vi "Swept H(f) from IIR cluster.vi"(6 "Sweep specs":T2={"Fstart"=1e-06, "Fstop"=0.4, "# points"=100, "type"=1} {"type" items=["linear", "exponential"]; "Fstop" format="%.2p"; "Fstart" format="%.2p"}, 9 "Fs":dbl=1.0 format="%.3p", 11 "IIR Filter Cluster":T1 {"Forward Coefficients" format="%.4f"; "Reverse Coefficients" format="%.4f"}) -> (2 "Phase (degrees)":cluster{dbl[], dbl[]}(graph)={[1e-06, 1.1391645578553926e-06, 1.2976958898738721e-06, 1.47828916461893e-06, 1.684014622595541e-06, 1.9183697729710654e-06, 2.1853388542297337e-06, 2.489460569642825e-06, 2.8359052491156023e-06, 3.230562749228562e-06, 3.6801425858490564e-06, 4.1922880016535415e-06, 4.775705907806124e-06, 5.440314908913349e-06, 6.197413927806377e-06, 7.059874296916403e-06, 8.042358581961425e-06, 9.161569858134609e-06, 1.0436535676703204e-05, 1.1888931549693636e-05, 1.3543449452179778e-05, 1.5428217607029237e-05, 1.7575278688808244e-05, 2.002113457672155e-05, 2.2807366917854315e-05, 2.598134405082322e-05, 2.9597026308144866e-05, 3.371588338815227e-05, 3.840793939256846e-05, 4.3752963296271964e-05, 4.984182508826087e-05, 5.6778040639374506e-05, 6.467953156084857e-05, 7.368062997280797e-05, 8.393436226548058e-05, 9.561505067903054e-05, 0.00010892127693109878, 0.00012407925827625992, 0.0001413466933933007, 0.0001610171434837011, 0.0001834250230637487, 0.00020895128529803048, 0.0002380298985298469, 0.000271155224115117, 0.00030889042098927716, 0.000351877019852016, 0.000400845829739195, 0.00045662936240302806, 0.0005201759857256353, 0.0005925660467861364, 0.0006750302386872469, 0.0007689705233931778, 0.0008759839662850192, 0.000997889887641487, 0.001136760792643482, 0.0012949576057390579, 0.0014751698083832116, 0.0016804611625284855, 0.0019143217972049213, 0.002180727543705885, 0.0024842075281287907, 0.002829921170401872, 0.0032237458988464635, 0.0036723770714975667, 0.004183441802930807, 0.004765628631749439, 0.005428835233189849, 0.006184336688086492, 0.007044977168912931, 0.008025388301726034, 0.009142237916353577, 0.010414513413791729, 0.01186384456830111, 0.013514871252113834, 0.015395662334386813, 0.017538192876042673, 0.01997888773321975, 0.022759240811055802, 0.02592652049565079, 0.029534573257156804, 0.03364473908593674, 0.038326894324991166, 0.043660639627698915, 0.04973665323717127, 0.056658232594129186, 0.06454305048195917, 0.0735251555649193, 0.08375725133036026, 0.09541329217893284, 0.10869144079854141, 0.123817437099936, 0.14104843598873648, 0.16067737921930364, 0.18303797565572127, 0.20851037460859584, 0.23752762869926336, 0.2705830561256362, 0.30823862749452124, 0.3511345198037494, 0.40000000000000374], [-1.9375458649467934, -2.206420614039625, -2.512349605053203, -2.860316782462487, -3.2559181849934364, -3.7054091499612234, -4.21574082276718, -4.794577025773823, -5.450278424878941, -6.191835453674648, -7.028724507250726, -7.970653736952076, -9.027156331264258, -10.206982762762935, -11.517243576328537, -12.9622682973866, -14.542184402441919, -16.251294530613507, -18.076446778055725, -19.99574219328411, -21.97806486554142, -23.983974500130337, -25.96836944127362, -27.884943680286753, -29.691867439660662, -31.357509793883324, -32.86468078379547, -34.21203701438905, -35.41200912612372, -36.48566534908234, -37.455944713890034, -38.341281611044664, -39.15155180775962, -39.88750210607899, -40.543640220832486, -41.113376045518294, -41.594444666033596, -41.9925811703799, -42.32208102040144, -42.6030285269283, -42.856196280103276, -43.09747087910708, -43.33383712202392, -43.56239072935225, -43.77275390492707, -43.95203592905604, -44.09055837692053, -44.1862863529227, -44.24637478614913, -44.285282336320996, -44.32014685127728, -44.36510689103546, -44.426634567539026, -44.501577299794185, -44.57862385087098, -44.64266924284485, -44.680502357974596, -44.68575986661503, -44.661355232192065, -44.61850540966146, -44.57270899214032, -44.53813286423849, -44.522440426494676, -44.523933722993824, -44.532042847954976, -44.530983308954184, -44.505254096957685, -44.44498145206778, -44.34916836352415, -44.22566764157143, -44.087881722818125, -43.94937644139832, -43.81835048285295, -43.6939531036865, -43.56577140029595, -43.41665885915146, -43.227865076298286, -42.98459058766059, -42.679934077247935, -42.315778839892594, -41.90027049475206, -41.44276843348109, -40.94806443905276, -40.41192286426785, -39.81951267901921, -39.147248640441994, -38.36731824622104, -37.453191443507, -36.38404639137267, -35.14642919371123, -33.732458269032456, -32.135124592057934, -30.34227788632209, -28.331347333992532, -26.066552278969493, -23.499412451363234, -20.572098548544368, -17.222013665578167, -13.385367266066789, -8.997654066440159]}, 3 "Magnitude (dB)":cluster{dbl[], dbl[]}(graph)={[1e-06, 1.1391645578553926e-06, 1.2976958898738721e-06, 1.47828916461893e-06, 1.684014622595541e-06, 1.9183697729710654e-06, 2.1853388542297337e-06, 2.489460569642825e-06, 2.8359052491156023e-06, 3.230562749228562e-06, 3.6801425858490564e-06, 4.1922880016535415e-06, 4.775705907806124e-06, 5.440314908913349e-06, 6.197413927806377e-06, 7.059874296916403e-06, 8.042358581961425e-06, 9.161569858134609e-06, 1.0436535676703204e-05, 1.1888931549693636e-05, 1.3543449452179778e-05, 1.5428217607029237e-05, 1.7575278688808244e-05, 2.002113457672155e-05, 2.2807366917854315e-05, 2.598134405082322e-05, 2.9597026308144866e-05, 3.371588338815227e-05, 3.840793939256846e-05, 4.3752963296271964e-05, 4.984182508826087e-05, 5.6778040639374506e-05, 6.467953156084857e-05, 7.368062997280797e-05, 8.393436226548058e-05, 9.561505067903054e-05, 0.00010892127693109878, 0.00012407925827625992, 0.0001413466933933007, 0.0001610171434837011, 0.0001834250230637487, 0.00020895128529803048, 0.0002380298985298469, 0.000271155224115117, 0.00030889042098927716, 0.000351877019852016, 0.000400845829739195, 0.00045662936240302806, 0.0005201759857256353, 0.0005925660467861364, 0.0006750302386872469, 0.0007689705233931778, 0.0008759839662850192, 0.000997889887641487, 0.001136760792643482, 0.0012949576057390579, 0.0014751698083832116, 0.0016804611625284855, 0.0019143217972049213, 0.002180727543705885, 0.0024842075281287907, 0.002829921170401872, 0.0032237458988464635, 0.0036723770714975667, 0.004183441802930807, 0.004765628631749439, 0.005428835233189849, 0.006184336688086492, 0.007044977168912931, 0.008025388301726034, 0.009142237916353577, 0.010414513413791729, 0.01186384456830111, 0.013514871252113834, 0.015395662334386813, 0.017538192876042673, 0.01997888773321975, 0.022759240811055802, 0.02592652049565079, 0.029534573257156804, 0.03364473908593674, 0.038326894324991166, 0.043660639627698915, 0.04973665323717127, 0.056658232594129186, 0.06454305048195917, 0.0735251555649193, 0.08375725133036026, 0.09541329217893284, 0.10869144079854141, 0.123817437099936, 0.14104843598873648, 0.16067737921930364, 0.18303797565572127, 0.20851037460859584, 0.23752762869926336, 0.2705830561256362, 0.30823862749452124, 0.3511345198037494, 0.40000000000000374], [40.53447659163172, 40.53180177091481, 40.52833432686184, 40.52384078879847, 40.51801987030083, 40.51048341660593, 40.500732435641986, 40.48812724096096, 40.471850753943734, 40.4508642162466, 40.42385509599218, 40.38917804456189, 40.34479166378482, 40.28819691670524, 40.21638755890904, 40.1258290199095, 40.01248909094065, 39.87194967026278, 39.69962992234827, 39.491141938524756, 39.242774546341295, 38.95205732123354, 38.618302589068534, 38.24297866393063, 37.82976148053271, 37.38416635600529, 36.91277442379043, 36.422204988307804, 35.918091405997636, 35.404345091743956, 34.88291961256761, 34.354133589587775, 33.8174295546657, 33.27230158815923, 32.71907095039404, 32.15924702123769, 31.595361306885795, 31.030351846440382, 30.46673611295985, 29.905884771665182, 29.347669952181615, 28.790624104323644, 28.23255884240186, 27.67142516214559, 27.10610788431204, 26.53687004245427, 25.965288918373965, 25.39370897898882, 24.824411480737815, 24.25880270538491, 23.696915766451212, 23.137407191388665, 22.578050099193895, 22.016545785965008, 21.45136016225443, 20.882282414719292, 20.310503752392446, 19.73818787407076, 19.167688873919033, 18.60069991853496, 18.037641061309426, 17.47750799114926, 16.918236567839475, 16.357451150553178, 15.793325762787306, 15.225246305860107, 14.654034044427366, 14.081649479043161, 13.510483966391678, 12.942495749414242, 12.378503397049617, 11.817892725603942, 11.258843599609207, 10.698994750605511, 10.136306216446753, 9.569807594308964, 8.999961770502013, 8.428513209001983, 7.857876845809001, 7.2902903372401875, 6.727038483079895, 6.168033071996821, 5.61190342530427, 5.0565688412062935, 4.500090793124011, 3.9415030197140433, 3.3813276559239673, 2.8216018301149126, 2.2654198880086147, 1.7161763255313247, 1.1768087489521042, 0.6493480074874463, 0.13498205146464481, -0.36533130736345204, -0.8498452795404117, -1.3148564742385251, -1.7536494487710232, -2.1556864804557736, -2.5059280952335254, -2.7838160888419043]})   [LabVIEW 2010, in "NI_AALBase.lvlib"]
uses:
  NI_AALBase.lvlib
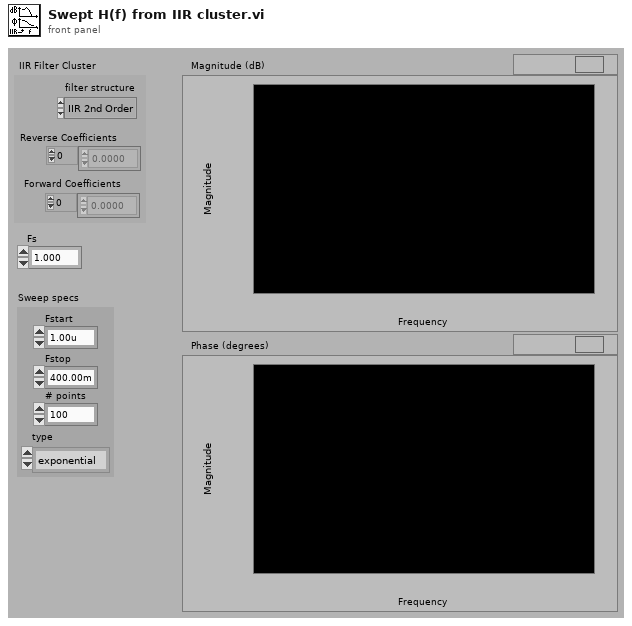
[diagram p1: front panel]
types:
  T1 = cluster{"filter structure":enum32{"IIR 2nd Order", "IIR 4th Order"}, "Reverse Coefficients":dbl[], "Forward Coefficients":dbl[]}
  T2 = cluster{"Fstart":dbl, "Fstop":dbl, "# points":i32, "type":u16}
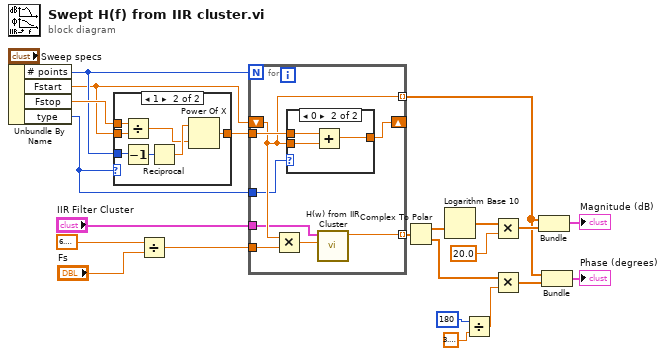
[diagram p0: block diagram]
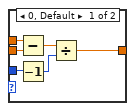
[diagram p2: hidden frame]
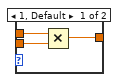
[diagram p3: hidden frame]
diagram:
  n1 = Unbundle By Name("Sweep specs") -> ("# points"=w12:i32, "Fstart"=w6:dbl, "Fstop"=w13:dbl, "type"=w7:u16)
  n2 = case shown="1" w7 {
    tunnel: w13 -> [w28 w35]
    tunnel: w6 -> [w29 w36]
    tunnel: w12 -> [w25 w34]
    tunnel: [w24 w30] -> w11
    frame 0, Default {
      n3 = Subtract(x=w28, y=w29) -> (x-y=w27:dbl)
      n4 = Decrement(x=w25) -> (x-1=w26:i32)
      n5 = Divide(x=w27, y=w26) -> (x/y=w24:dbl)
    }
    frame 1 {
      n6 = Divide(x=w35, y=w36) -> (x/y=w31:dbl)
      n7 = Decrement(x=w34) -> (x-1=w33:i32)
      n8 = Reciprocal(x=w33) -> (1/x=w32:dbl)
      n9 = Power Of X(1:w31, 2:w32) -> (0:w30:dbl)
    }
  }
  n10 = Divide(x=6.283185307179586, y="Fs") -> (x/y=w8:dbl)
  n11 = for {
    N: w12 -> [_]
    tunnel: [w42] -> w15 mode=indexing
    shift-left: w6 -> [w42]
    shift-right: [w44] -> _
    tunnel: w11 -> [w43]
    tunnel: w8 -> [w41]
    tunnel: w7 -> [w40]
    tunnel: "IIR Filter Cluster" -> [w38]
    tunnel: [w37] -> w2 mode=indexing
    n12 = Multiply(x=w42, y=w41) -> (x*y=w39:dbl)
    n13 = case shown="0" w40 {
      tunnel: [w47 w50] -> w44
      tunnel: w43 -> [w46 w49]
      tunnel: w42 -> [w45 w48]
      frame 1, Default {
        n14 = Multiply(x=w46, y=w45) -> (x*y=w47:dbl)
      }
      frame 0 {
        n15 = Add(x=w49, y=w48) -> (x+y=w50:dbl)
      }
    }
    n16 = call "H(w) from IIR Cluster.vi"("w"=w39, "IIR Filter Cluster"=w38) -> ("Complex response"=w37:cdb)  [unwired: 9 in]
  }
  n17 = Complex To Polar(r * e^(i*theta)=w2) -> (r=w23:dbl[], theta=w1:dbl[])
  n18 = Logarithm Base 10(1:w23) -> (0:w5:dbl[])
  n19 = Divide(x=180, y=3.141592653589793) -> (x/y=w17:dbl)
  n20 = Multiply(x=w5, y=20.0) -> (x*y=w21:dbl[])
  n21 = Multiply(x=w1, y=w17) -> (x*y=w14:dbl[])
  n22 = Bundle(w15, w21) -> (→"Magnitude (dB)":cluster{dbl[], dbl[]})  [unwired: 1 in]
  n23 = Bundle(w15, w14) -> (→"Phase (degrees)":cluster{dbl[], dbl[]})  [unwired: 1 in]
